vi "USER_EDITOR_prepare_INSERT_statement.vi"(8 "error_in":errorcluster, 10 "selected_record":i32, 11 "USER_EDIT_records":string[][](array[string])) -> (0 "error_out":errorcluster, 3 "INSERT_statement":string)   [LabVIEW 2019]
uses:
  FGV/USER_EDITOR_records_display/FGV_USER_EDITOR_records_display.ctl
  <userlib>/_OpenG.lib/array/array.llb/Filter 1D Array (String)__ogtk.vi
  <userlib>/_OpenG.lib/array/array.llb/Delete Elements from 1D Array (String)__ogtk.vi
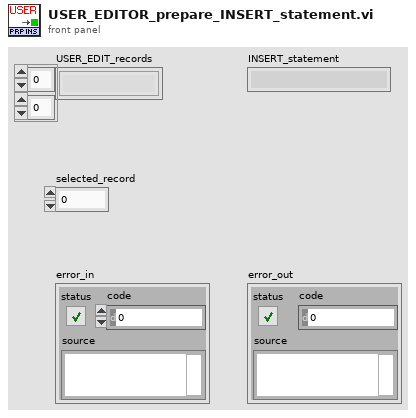
[diagram p1: front panel]
types:
  T1 = typedef "FGV_USER_EDITOR_records_display.ctl" = enum16{"initialize", "set_user_edit_tables_names", "set_headers", "set_records", "get_user_edit_table_name", "get_user_edit_hist_table_name", "get_headers", "get_uneditable_columns", "get_all_info", "record_added?", "record_inserted?", "record_edited?", "record_updated?", "record_deleted?", "discard_changes"}
  T2 = typedef "USER_EDITOR_all_info.ctl" = cluster{"user_table":string, "user_history":string, "headers":string[], "uneditable_columns":string[], "uneditable_columns":i32[], "editable_columns":i32[], "values_in_database":string[][], "size":cluster{"columns":i32, "SQL_rows":i32, "disp_rows":i32}, "USER_record_states":T3[]}
  T3 = typedef "SQL_record_states.ctl" = enum16{"Equal", "Added", "Edited", "Deleted"}
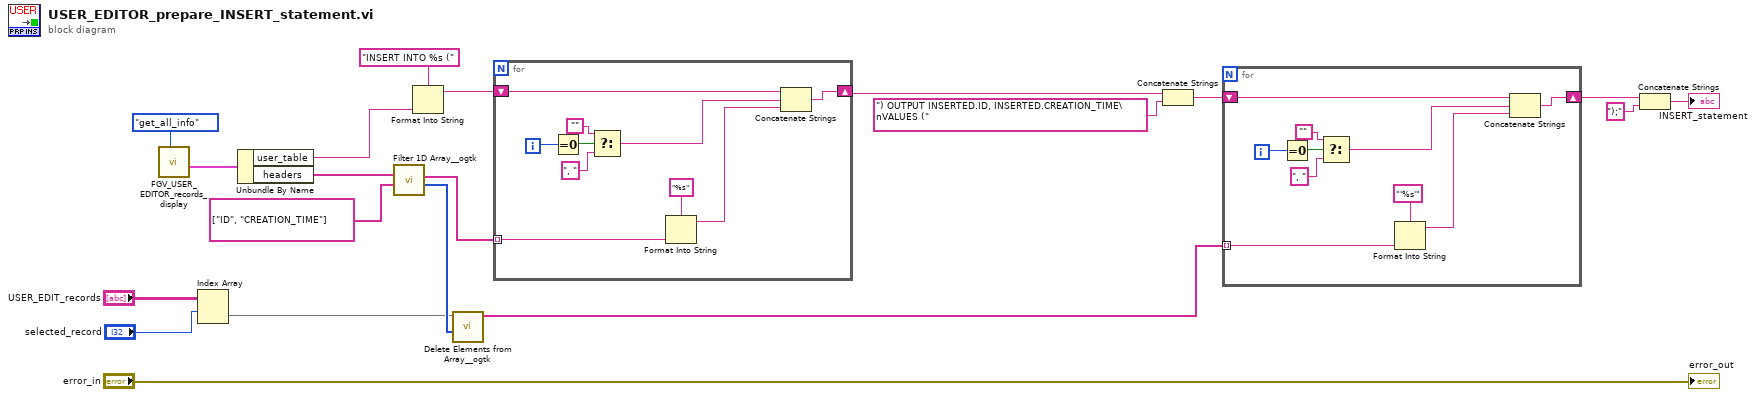
[diagram p0: block diagram]
diagram:
  n1 = call "FGV_USER_EDITOR_records_display.vi"("options"=FGV_USER_EDITOR_records_display."get_all_info") -> ("all_info"=w1:T2)  [unwired: 7 in, 3 out]
  n2 = Index Array(array="USER_EDIT_records", index (row)="selected_record") -> (element=w3:string[])  [unwired: 1 in]
  n3 = Unbundle By Name(w1) -> ("user_table"=w6:string, "headers"=w7:string[])
  n4 = call-poly <userlib>:"Filter 1D Array__ogtk.vi"("items to filter"=string[] ["ID", "CREATION_TIME"], "array"=w7) -> ("filtered item indices"=w12:i32[], "filtered array"=w14:string[])  [unwired: 4 in]
  n5 = Format Into String(format string="INSERT INTO %s (", w6) -> (resulting string=w17:string)  [unwired: 2 in, 1 out]
  n6 = call-poly <userlib>:"Delete Elements from Array__ogtk.vi"("indices"=w12, "array"=w3) -> ("array w/ subset deleted"=w11:string[])  [unwired: 8 in, 1 out]
  n7 = for {
    tunnel: w14 -> [w23] mode=indexing
    shift-right: [w25] -> w20
    shift-left: w17 -> [w26]
    i -> [w30]
    n8 = Equal To 0?(x=w30) -> (x = 0?=w29:bool)
    n9 = Select(t="", s=w29, f=", ") -> (s? t:f=w24:string)
    n10 = Format Into String(format string="%s", w23) -> (resulting string=w22:string)  [unwired: 2 in, 1 out]
    n11 = Concatenate Strings(w26, w24, w22) -> (w25:string)
  }
  n12 = Concatenate Strings(w20, ") OUTPUT INSERTED.ID, INSERTED.CREATION_TIME\nVALUES (" ("string")) -> (w13:string)
  n13 = for {
    tunnel: w11 -> [w33] mode=indexing
    shift-right: [w35] -> w9
    shift-left: w13 -> [w36]
    i -> [w40]
    n14 = Equal To 0?(x=w40) -> (x = 0?=w39:bool)
    n15 = Select(t="", s=w39, f=", ") -> (s? t:f=w34:string)
    n16 = Format Into String(format string="'%s'", w33) -> (resulting string=w32:string)  [unwired: 2 in, 1 out]
    n17 = Concatenate Strings(w36, w34, w32) -> (w35:string)
  }
  n18 = Concatenate Strings(w9, ");" ("string")) -> (→"INSERT_statement":string)
  "error_out" <- "error_in"
